vi "ToggleAllRooms.vi"(0 "reference in":refnum<class "HeatingSystem.lvclass">, 5 "Error In":errorcluster) -> (14 "reference out":refnum<class "HeatingSystem.lvclass">, 19 "Error Out":errorcluster)   [LabVIEW 2024, in "HeatingSystem.lvclass"]
doc: "Toggle all of the elements in all of the rooms"
uses:
  HeatingSystem.lvclass
  HeatingSystem.lvclass/HeatingSystem.ctl
panel:
  # "Connector Pane"
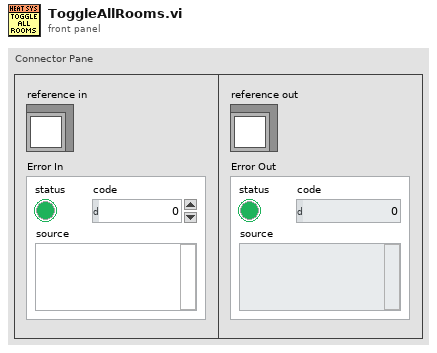
[diagram p1: front panel]
types:
  T1 = typedef "HeatingSystem.lvclass/ObjectAttributes.ctl" = cluster{"Rooms":T2}
  T2 = typedef "Rooms Map.ctl" = map{string, refnum<class "Room.lvclass">}
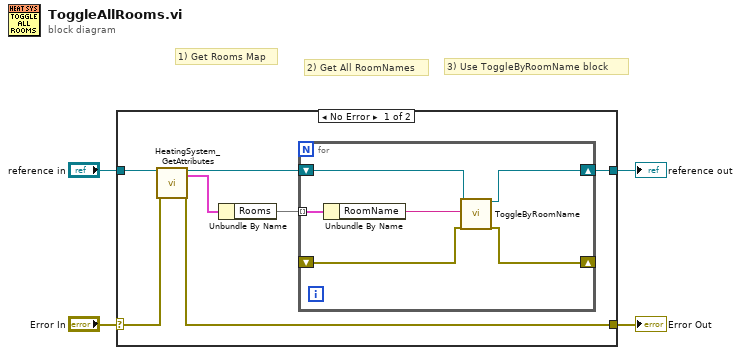
[diagram p0: block diagram]
diagram:
  # "3) Use ToggleByRoomName block"
  # "2) Get All RoomNames"
  # "1) Get Rooms Map"
  n1 = case shown="No Error" "Error In" {
    selector: "Error In" -> [w11 w19]
    tunnel: [w9 w19] -> w3
    tunnel: [w5 w18] -> w1
    tunnel: "reference in" -> [w8 w18]
    frame No Error {
      n2 = call "HeatingSystem_GetAttributes.vi"("reference in"=w8, "Error In"=w11) -> ("reference out"=w6:refnum<class "HeatingSystem.lvclass">, "Data"=w10:T1, "Error Out"=w9:errorcluster)  [unwired: 14 in, 1 out]
      n3 = Unbundle By Name(w10) -> ("Rooms"=w7:T2)
      n4 = for {
        tunnel: w7 -> [w17] mode=indexing
        shift-right: [w13] -> w5
        shift-left: w6 -> [w16]
        shift-right: [w12] -> _
        shift-left: _ -> [w15]
        n5 = Unbundle By Name(w17) -> ("RoomName"=w14:string)
        n6 = call-dynamic "ToggleByRoomName.vi"("reference in"=w16, "RoomName"=w14, "Error In"=w15) -> ("reference out"=w13:refnum<class "HeatingSystem.lvclass">, "Error Out"=w12:errorcluster)  [unwired: 15 in]
      }
    }
    frame Error {
    }
  }
  "Error Out" <- w3
  "reference out" <- w1
